vi "Day02-06_디버깅.vi"() -> ()   [LabVIEW 2021]
panel:
  out "숫자형":i32
  out "숫자(0에서 1)":dbl
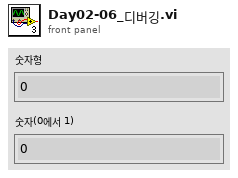
[diagram p1: front panel]
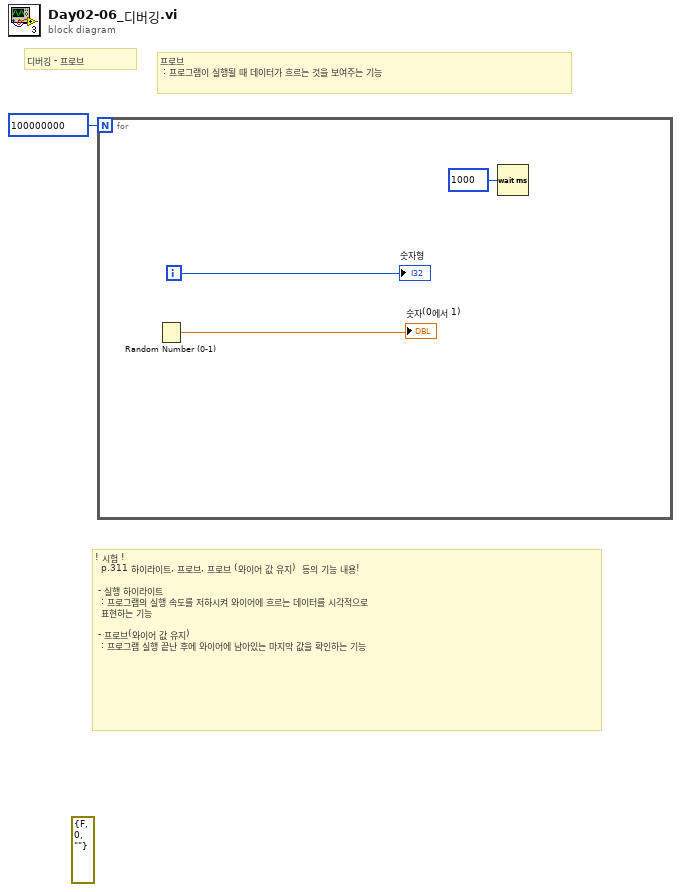
[diagram p0: block diagram]
diagram:
  (unwired) errorcluster {"status"=FALSE, "code"=0, "source"=""} ("에러 상수")
  # "! 시험 !\n  p.311 하이라이트, 프로브, 프로브 (와이어 값 유지)  등의 기능 내용!\n\n - 실행 하이라이트 \n  : 프로그램의 실행 속도를 저하시켜 와이어에 흐르는 데이터를 시각적으로\n  표현하는 기능\n\n - 프로브(와이어 값 유지) \n  : 프로그램 실행 끝난 후에 와이어에 남아있는 마지막 값을 확인하는 기능"
  # "프로브 \n : 프로그램이 실행될 때 데이터가 흐르는 것을 보여주는 기능"
  # "디버깅 - 프로브"
  n1 = for {
    N: 100000000 -> [_]
    i -> [w3]
    n2 = Random Number (0-1)() -> (number: 0 to 1=→"숫자(0에서 1)":dbl)
    n3 = Wait (ms)(milliseconds to wait=u32 1000 ("대기 시간 (ms)")) -> ()  [unwired: 1 out]
    "숫자형" <- w3
  }
